vi "measureDelayBetweenChannels.vi"(7 "Measurement time (s)":dbl=2.0 caption="Delay Time (s)", 8 "error in (no error)":errorcluster, 9 "channel_2":i32=2, 10 "channel_1":i32=1, 11 "TimeTagger ref in":refnum<k24>) -> (0 "error out":errorcluster, 2 "measured delay, ps":i64, 3 "TimeTagger ref out":refnum<k24>)   [LabVIEW 2014]
doc: "This code uses Correlation measurement \nto determine propagation delay between two correlated signals."
uses:
  SwabianInstruments.TimeTagger
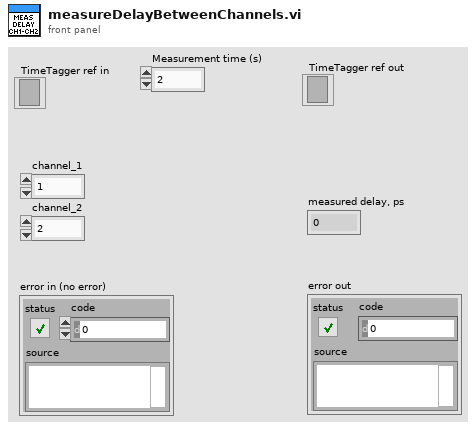
[diagram p1: front panel]
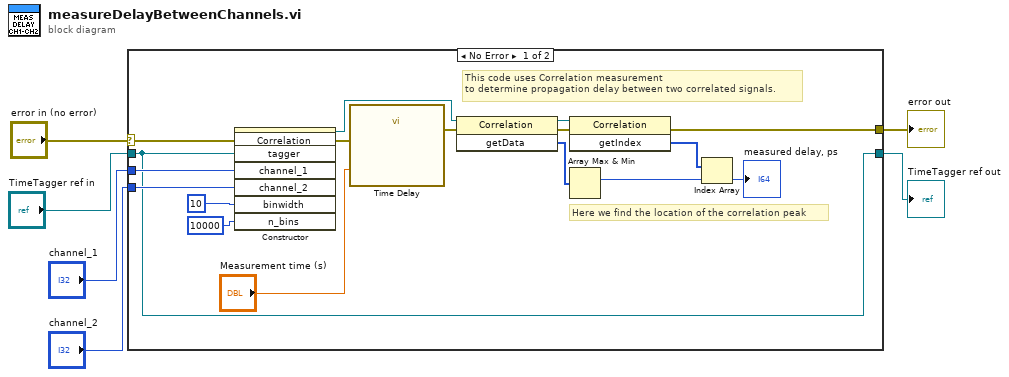
[diagram p0: block diagram]
diagram:
  n1 = case shown="No Error" "error in (no error)" {
    selector: "error in (no error)" -> [w23 w24]
    tunnel: "channel_2" -> [w13 _]
    tunnel: "channel_1" -> [w12 _]
    tunnel: "TimeTagger ref in" -> [w7 w25]
    tunnel: [w8 w24] -> w2
    tunnel: [w7 w25] -> w1
    frame No Error {
      # "Here we find the location of the correlation peak"
      # "This code uses Correlation measurement \nto determine propagation delay between two correlated signals."
      n2 = constructor class="Correlation"(error in=w23, "tagger"=w7, "channel_1"=w12, "channel_2"=w13, "binwidth"=i64 10, "n_bins"=10000) -> (reference out=w18:refnum<k24>, error out=w17:errorcluster)  [unwired: 2 in, 6 out]
      n3 = call "Time Delay"("error in (no error)"=w17, "Delay Time (s)"="Measurement time (s)") -> ("error out"=w16:errorcluster)  [unwired: 9 in]
      n4 = invoke class="Correlation" method="getData"(reference=w18, error in=w16) -> (reference out=w10:refnum<k24>, error out=w11:errorcluster, "getData"=w19:i32[])  [unwired: 1 in]
      n5 = invoke class="Correlation" method="getIndex"(reference=w10, error in=w11) -> (error out=w8:errorcluster, "getIndex"=w21:i64[])  [unwired: 1 in, 1 out]
      n6 = Array Max & Min(array=w19) -> (max index (indices)=w20:i32)  [unwired: 3 out]
      n7 = Index Array(array=w21, index=w20) -> (element=→"measured delay, ps":i64)
    }
    frame Error {
    }
  }
  "error out" <- w2
  "TimeTagger ref out" <- w1
